vi "VI tree.vi"   [LabVIEW 2019]
uses:
  <vilib>/addons/control/pid/NI_PID_pid.lvlib
  <vilib>/addons/control/pid/pid.llb/PID (DBL).vi
panel:
  # "Ybbaek.  ALL RIGHTS RESERVED.\n- RLmodel"
  # "SEE DIAGRAM\nFOR VI Tree"
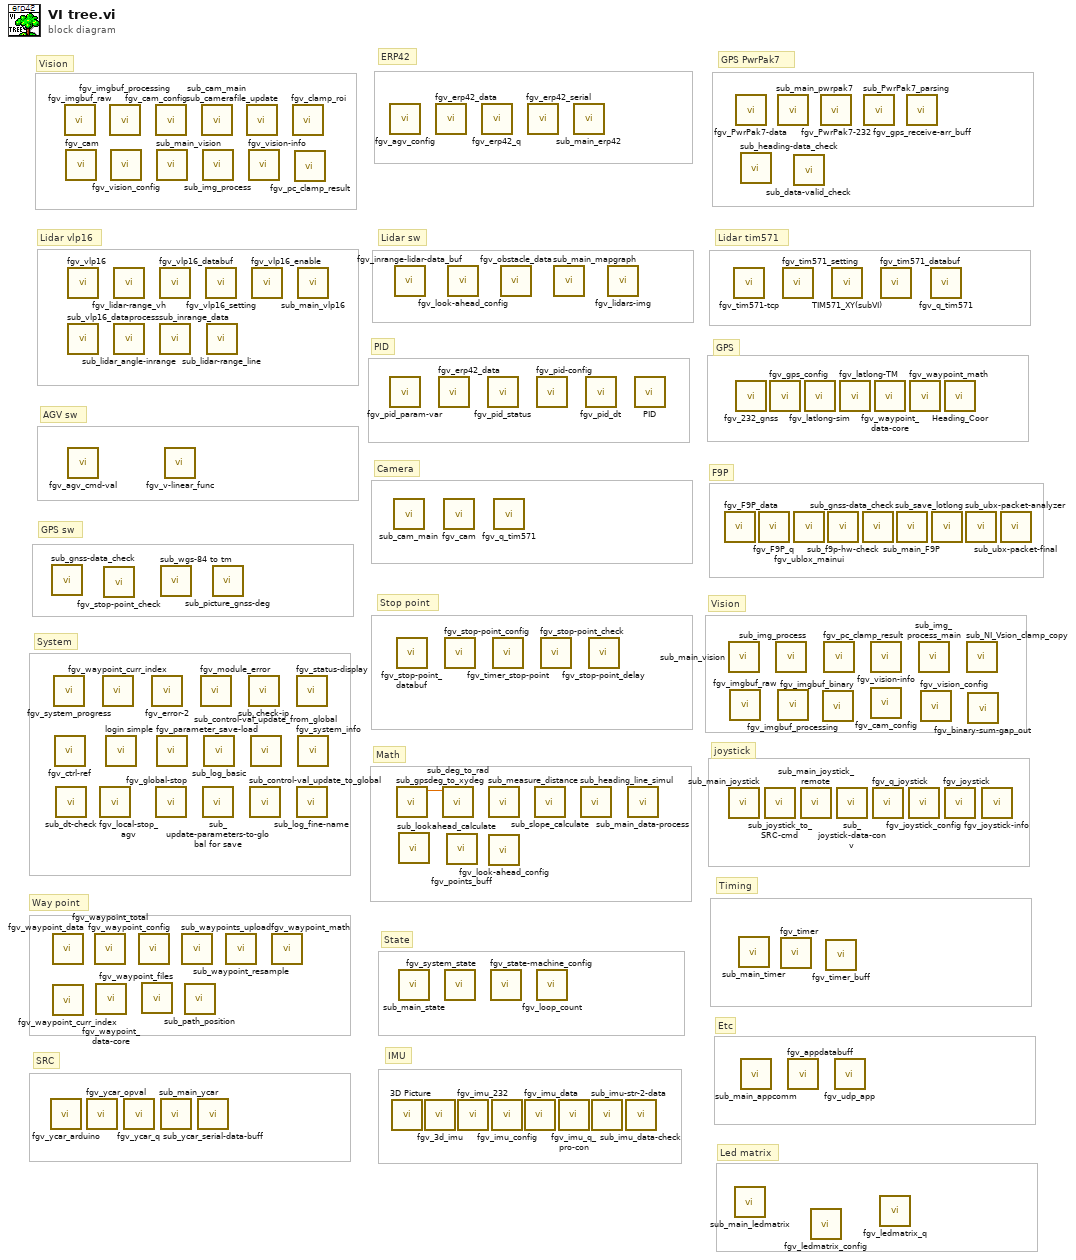
[diagram p0: block diagram]
diagram:
  # "Led matrix"
  # "SRC"
  # "F9P"
  # "joystick"
  # "Etc"
  # "ERP42"
  # "Timing"
  # "Vision"
  # "Camera"
  # "IMU"
  # "GPS sw"
  # "GPS"
  # "Lidar tim571"
  # "Stop point"
  # "GPS PwrPak7"
  # "State"
  # "System"
  # "Way point"
  # "Math"
  # "AGV sw"
  # "PID"
  # "Lidar sw"
  # "Lidar vlp16"
  # "Vision"
  n1 = call "fgv_ycar_arduino.vi"() -> ()  [unwired: 9 in, 3 out]
  n2 = call "sub_gnss-data_check.vi"() -> ()  [unwired: 9 in, 3 out]
  n3 = call "fgv_waypoint_data.vi"() -> ()  [unwired: 9 in, 3 out]
  n4 = call "fgv_waypoint_curr_index.vi"() -> ()  [unwired: 11 in, 1 out]
  n5 = call "fgv_system_progress.vi"() -> ()  [unwired: 11 in, 1 out]
  n6 = call "fgv_ctrl-ref.vi"() -> ()  [unwired: 10 in, 2 out]
  n7 = call "sub_dt-check.vi"() -> ()  [unwired: 10 in, 2 out]
  n8 = call "fgv_imgbuf_raw.vi"() -> ()  [unwired: 10 in, 2 out]
  n9 = call "fgv_cam.vi"() -> ()  [unwired: 9 in, 3 out]
  n10 = call "fgv_vlp16.vi"() -> ()  [unwired: 10 in, 2 out]
  n11 = call "sub_vlp16_dataprocess.vi"() -> ()  [unwired: 10 in, 2 out]
  n12 = call "fgv_agv_cmd-val.vi"() -> ()  [unwired: 10 in, 2 out]
  n13 = call "fgv_ycar_opval.vi"() -> ()  [unwired: 11 in, 1 out]
  n14 = call "fgv_waypoint_total.vi"() -> ()  [unwired: 11 in, 1 out]
  n15 = call "fgv_waypoint_data-core.vi"() -> ()  [unwired: 11 in, 1 out]
  n16 = call "fgv_local-stop_agv.vi"() -> ()  [unwired: 11 in, 1 out]
  n17 = call "fgv_waypoint_curr_index.vi"() -> ()  [unwired: 11 in, 1 out]
  n18 = call "fgv_stop-point_check.vi"() -> ()  [unwired: 11 in, 1 out]
  n19 = call "login simple.vi"() -> ()  [unwired: 11 in, 1 out]
  n20 = call "fgv_imgbuf_processing.vi"() -> ()  [unwired: 10 in, 2 out]
  n21 = call "fgv_vision_config.vi"() -> ()  [unwired: 10 in, 2 out]
  n22 = call "fgv_lidar-range_vh.vi"() -> ()  [unwired: 11 in, 1 out]
  n23 = call "sub_lidar_angle-inrange.vi"() -> ()  [unwired: 9 in, 3 out]
  n24 = call "fgv_ycar_q.vi"() -> ()  [unwired: 10 in, 2 out]
  n25 = call "fgv_waypoint_config.vi"() -> ()  [unwired: 11 in, 1 out]
  n26 = call "fgv_waypoint_files.vi"() -> ()  [unwired: 10 in, 2 out]
  n27 = call "fgv_error-2.vi"() -> ()  [unwired: 10 in, 2 out]
  n28 = call "fgv_cam_config.vi"() -> ()  [unwired: 11 in, 1 out]
  n29 = call "fgv_global-stop.vi"() -> ()  [unwired: 11 in, 1 out]
  n30 = call "sub_main_vision.vi"() -> ()  [unwired: 11 in, 1 out]
  n31 = call "fgv_parameter_save-load.vi"() -> ()  [unwired: 10 in, 2 out]
  n32 = call "fgv_vlp16_databuf.vi"() -> ()  [unwired: 9 in, 3 out]
  n33 = call "sub_inrange_data.vi"() -> ()  [unwired: 9 in, 3 out]
  n34 = call "sub_wgs-84 to tm.vi"() -> ()  [unwired: 11 in, 1 out]
  n35 = call "sub_main_ycar.vi"() -> ()  [unwired: 11 in, 1 out]
  n36 = call "fgv_v-linear_func.vi"() -> ()  [unwired: 11 in, 1 out]
  n37 = call "sub_waypoints_upload.vi"() -> ()  [unwired: 10 in, 2 out]
  n38 = call "sub_path_position.vi"() -> ()  [unwired: 12 in]
  n39 = call "sub_ycar_serial-data-buff.vi"() -> ()  [unwired: 10 in, 2 out]
  n40 = call "fgv_module_error.vi"() -> ()  [unwired: 9 in, 3 out]
  n41 = call "sub_cam_main.vi"() -> ()  [unwired: 11 in, 1 out]
  n42 = call "sub_img_process.vi"() -> ()  [unwired: 10 in, 2 out]
  n43 = call "sub_update-parameters-to-global for save.vi"() -> ()  [unwired: 12 in]
  n44 = call "sub_log_basic.vi"() -> ()  [unwired: 11 in, 1 out]
  n45 = call "fgv_vlp16_setting.vi"() -> ()  [unwired: 9 in, 3 out]
  n46 = call "sub_lidar-range_line.vi"() -> ()  [unwired: 11 in, 1 out]
  n47 = call "sub_picture_gnss-deg.vi"() -> ()  [unwired: 11 in, 1 out]
  n48 = call "sub_waypoint_resample.vi"() -> ()  [unwired: 10 in, 2 out]
  n49 = call "sub_camerafile_update.vi"() -> ()  [unwired: 12 in]
  n50 = call "fgv_vision-info.vi"() -> ()  [unwired: 11 in, 1 out]
  n51 = call "sub_check-ip.vi"() -> ()  [unwired: 10 in, 2 out]
  n52 = call "sub_control-val_update_to_global.vi"() -> ()  [unwired: 12 in]
  n53 = call "sub_control-val_update_from_global.vi"() -> ()  [unwired: 12 in]
  n54 = call "fgv_vlp16_enable.vi"() -> ()  [unwired: 11 in, 1 out]
  n55 = call "fgv_waypoint_math.vi"() -> ()  [unwired: 10 in, 2 out]
  n56 = call "fgv_clamp_roi.vi"() -> ()  [unwired: 11 in, 1 out]
  n57 = call "fgv_pc_clamp_result.vi"() -> ()  [unwired: 8 in, 4 out]
  n58 = call "fgv_status-display.vi"() -> ()  [unwired: 11 in, 1 out]
  n59 = call "sub_log_fine-name.vi"() -> ()  [unwired: 11 in, 1 out]
  n60 = call "sub_main_vlp16.vi"() -> ()  [unwired: 11 in, 1 out]
  n61 = call "fgv_system_info.vi"() -> ()  [unwired: 11 in, 1 out]
  n62 = call "fgv_agv_config.vi"() -> ()  [unwired: 10 in, 2 out]
  n63 = call "fgv_pid_param-var.vi"() -> ()  [unwired: 11 in, 1 out]
  n64 = call "3D Picture.vi"() -> ()  [unwired: 12 in]
  n65 = call "sub_cam_main.vi"() -> ()  [unwired: 11 in, 1 out]
  n66 = call "fgv_inrange-lidar-data_buf.vi"() -> ()  [unwired: 10 in, 2 out]
  n67 = call "fgv_stop-point_databuf.vi"() -> ()  [unwired: 10 in, 2 out]
  n68 = call "sub_gpsdeg_to_xydeg.vi"() -> ("deg"=w1:dbl)  [unwired: 11 in]
  n69 = call "sub_lookahead_calculate.vi"() -> ()  [unwired: 7 in, 5 out]
  n70 = call "sub_main_state.vi"() -> ()  [unwired: 11 in, 1 out]
  n71 = call "fgv_3d_imu.vi"() -> ()  [unwired: 12 in]
  n72 = call "fgv_erp42_data.vi"() -> ()  [unwired: 9 in, 3 out]
  n73 = call "fgv_erp42_data.vi"() -> ()  [unwired: 9 in, 3 out]
  n74 = call "sub_deg_to_rad.vi"("deg in"=w1) -> ()  [unwired: 10 in, 1 out]
  n75 = call "fgv_cam.vi"() -> ()  [unwired: 9 in, 3 out]
  n76 = call "fgv_stop-point_config.vi"() -> ()  [unwired: 11 in, 1 out]
  n77 = call "fgv_system_state.vi"() -> ()  [unwired: 10 in, 2 out]
  n78 = call "fgv_points_buff.vi"() -> ()  [unwired: 7 in, 5 out]
  n79 = call "fgv_look-ahead_config.vi"() -> ()  [unwired: 11 in, 1 out]
  n80 = call "fgv_imu_232.vi"() -> ()  [unwired: 9 in, 3 out]
  n81 = call "fgv_erp42_q.vi"() -> ()  [unwired: 10 in, 2 out]
  n82 = call "fgv_pid_status.vi"() -> ()  [unwired: 9 in, 3 out]
  n83 = call "sub_measure_distance.vi"() -> ()  [unwired: 11 in, 1 out]
  n84 = call "fgv_look-ahead_config.vi"() -> ()  [unwired: 11 in, 1 out]
  n85 = call "fgv_state-machine_config.vi"() -> ()  [unwired: 11 in, 1 out]
  n86 = call "fgv_imu_config.vi"() -> ()  [unwired: 10 in, 2 out]
  n87 = call "fgv_timer_stop-point.vi"() -> ()  [unwired: 9 in, 3 out]
  n88 = call "fgv_q_tim571.vi"() -> ()  [unwired: 10 in, 2 out]
  n89 = call "fgv_obstacle_data.vi"() -> ()  [unwired: 8 in, 4 out]
  n90 = call "fgv_imu_data.vi"() -> ()  [unwired: 8 in, 4 out]
  n91 = call "fgv_erp42_serial.vi"() -> ()  [unwired: 8 in, 4 out]
  n92 = call "sub_slope_calculate.vi"() -> ()  [unwired: 9 in, 3 out]
  n93 = call "fgv_pid-config.vi"() -> ()  [unwired: 10 in, 2 out]
  n94 = call "fgv_loop_count.vi"() -> ()  [unwired: 10 in, 2 out]
  n95 = call "fgv_stop-point_check.vi"() -> ()  [unwired: 11 in, 1 out]
  n96 = call "sub_main_mapgraph.vi"() -> ()  [unwired: 11 in, 1 out]
  n97 = call "fgv_imu_q_pro-con.vi"() -> ()  [unwired: 10 in, 2 out]
  n98 = call "sub_main_erp42.vi"() -> ()  [unwired: 11 in, 1 out]
  n99 = call "sub_heading_line_simul.vi"() -> ()  [unwired: 10 in, 2 out]
  n100 = call "fgv_pid_dt.vi"() -> ()  [unwired: 11 in, 1 out]
  n101 = call "fgv_stop-point_delay.vi"() -> ()  [unwired: 10 in, 2 out]
  n102 = call "sub_imu-str-2-data.vi"() -> ()  [unwired: 10 in, 2 out]
  n103 = call "fgv_lidars-img.vi"() -> ()  [unwired: 11 in, 1 out]
  n104 = call "sub_imu_data-check.vi"() -> ()  [unwired: 11 in, 1 out]
  n105 = call "sub_main_data-process.vi"() -> ()  [unwired: 11 in, 1 out]
  n106 = call-poly <vilib>:"PID.vi"() -> ()  [unwired: 10 in, 2 out]
  n107 = call "fgv_F9P_data.vi"() -> ()  [unwired: 11 in, 1 out]
  n108 = call "sub_main_vision.vi"() -> ()  [unwired: 11 in, 1 out]
  n109 = call "sub_main_joystick.vi"() -> ()  [unwired: 11 in, 1 out]
  n110 = call "fgv_imgbuf_raw.vi"() -> ()  [unwired: 10 in, 2 out]
  n111 = call "fgv_tim571-tcp.vi"() -> ()  [unwired: 10 in, 2 out]
  n112 = call "sub_main_ledmatrix.vi"() -> ()  [unwired: 12 in]
  n113 = call "fgv_PwrPak7-data.vi"() -> ()  [unwired: 10 in, 2 out]
  n114 = call "fgv_232_gnss.vi"() -> ()  [unwired: 9 in, 3 out]
  n115 = call "sub_main_timer.vi"() -> ()  [unwired: 11 in, 1 out]
  n116 = call "sub_heading-data_check.vi"() -> ()  [unwired: 9 in, 3 out]
  n117 = call "sub_main_appcomm.vi"() -> ()  [unwired: 11 in, 1 out]
  n118 = call "fgv_F9P_q.vi"() -> ()  [unwired: 10 in, 2 out]
  n119 = call "sub_joystick_to_SRC-cmd.vi"() -> ()  [unwired: 10 in, 2 out]
  n120 = call "fgv_gps_config.vi"() -> ()  [unwired: 10 in, 2 out]
  n121 = call "sub_img_process.vi"() -> ()  [unwired: 10 in, 2 out]
  n122 = call "sub_main_pwrpak7.vi"() -> ()  [unwired: 11 in, 1 out]
  n123 = call "fgv_imgbuf_processing.vi"() -> ()  [unwired: 10 in, 2 out]
  n124 = call "fgv_timer.vi"() -> ()  [unwired: 9 in, 3 out]
  n125 = call "fgv_tim571_setting.vi"() -> ()  [unwired: 11 in, 1 out]
  n126 = call "fgv_appdatabuff.vi"() -> ()  [unwired: 11 in, 1 out]
  n127 = call "sub_data-valid_check.vi"() -> ()  [unwired: 9 in, 3 out]
  n128 = call "fgv_ublox_mainui.vi"() -> ()  [unwired: 11 in, 1 out]
  n129 = call "sub_main_joystick_remote.vi"() -> ()  [unwired: 11 in, 1 out]
  n130 = call "fgv_latlong-sim.vi"() -> ()  [unwired: 10 in, 2 out]
  n131 = call "fgv_ledmatrix_config.vi"() -> ()  [unwired: 11 in, 1 out]
  n132 = call "fgv_PwrPak7-232.vi"() -> ()  [unwired: 8 in, 4 out]
  n133 = call "fgv_imgbuf_binary.vi"() -> ()  [unwired: 10 in, 2 out]
  n134 = call "fgv_pc_clamp_result.vi"() -> ()  [unwired: 8 in, 4 out]
  n135 = call "fgv_timer_buff.vi"() -> ()  [unwired: 11 in, 1 out]
  n136 = call "sub_f9p-hw-check.vi"() -> ()  [unwired: 11 in, 1 out]
  n137 = call "TIM571_XY(subVI).vi"() -> ()  [unwired: 10 in, 2 out]
  n138 = call "fgv_udp_app.vi"() -> ()  [unwired: 10 in, 2 out]
  n139 = call "sub_joystick-data-conv.vi"() -> ()  [unwired: 10 in, 2 out]
  n140 = call "fgv_latlong-TM.vi"() -> ()  [unwired: 10 in, 2 out]
  n141 = call "sub_gnss-data_check.vi"() -> ()  [unwired: 9 in, 3 out]
  n142 = call "sub_PwrPak7_parsing.vi"() -> ()  [unwired: 11 in, 1 out]
  n143 = call "fgv_vision-info.vi"() -> ()  [unwired: 11 in, 1 out]
  n144 = call "fgv_cam_config.vi"() -> ()  [unwired: 11 in, 1 out]
  n145 = call "fgv_q_joystick.vi"() -> ()  [unwired: 10 in, 2 out]
  n146 = call "fgv_waypoint_data-core.vi"() -> ()  [unwired: 11 in, 1 out]
  n147 = call "fgv_ledmatrix_q.vi"() -> ()  [unwired: 10 in, 2 out]
  n148 = call "fgv_tim571_databuf.vi"() -> ()  [unwired: 9 in, 3 out]
  n149 = call "sub_main_F9P.vi"() -> ()  [unwired: 11 in, 1 out]
  n150 = call "fgv_gps_receive-arr_buff.vi"() -> ()  [unwired: 10 in, 2 out]
  n151 = call "fgv_joystick_config.vi"() -> ()  [unwired: 10 in, 2 out]
  n152 = call "fgv_waypoint_math.vi"() -> ()  [unwired: 10 in, 2 out]
  n153 = call "sub_img_process_main.vi"() -> ()  [unwired: 8 in, 4 out]
  n154 = call "fgv_vision_config.vi"() -> ()  [unwired: 10 in, 2 out]
  n155 = call "fgv_q_tim571.vi"() -> ()  [unwired: 10 in, 2 out]
  n156 = call "sub_save_lotlong.vi"() -> ()  [unwired: 12 in]
  n157 = call "Heading_Coor.vi"() -> ()  [unwired: 11 in, 1 out]
  n158 = call "fgv_joystick.vi"() -> ()  [unwired: 10 in, 2 out]
  n159 = call "sub_ubx-packet-analyzer.vi"() -> ()  [unwired: 9 in, 3 out]
  n160 = call "sub_NI_Vsion_clamp_copy.vi"() -> ()  [unwired: 7 in, 5 out]
  n161 = call "fgv_binary-sum-gap_out.vi"() -> ()  [unwired: 11 in, 1 out]
  n162 = call "fgv_joystick-info.vi"() -> ()  [unwired: 8 in, 4 out]
  n163 = call "sub_ubx-packet-final.vi"() -> ()  [unwired: 9 in, 3 out]
